vi "setEndTone.vi"(8 "error in (no error)":errorcluster, 10 "EndTone":refnum<class "ScriptEvent.lvclass">, 11 "SingleToneRamp.lvclass in":refnum<class "SingleToneRamp.lvclass">) -> (0 "error out":errorcluster, 3 "SingleToneRamp.lvclass out":refnum<class "SingleToneRamp.lvclass">)   [LabVIEW 2011, in "Tools.lvlib" / "Scripting.lvlib" / "SingleToneRamp.lvclass"]
uses:
  SingleToneRamp.lvclass
  ScriptEvent.lvclass
  SingleTone.lvclass
  SingleToneRamp.lvclass/SingleToneRamp.ctl
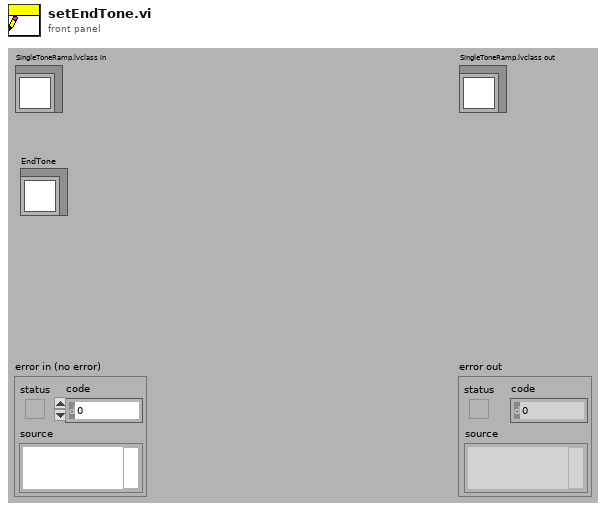
[diagram p1: front panel]
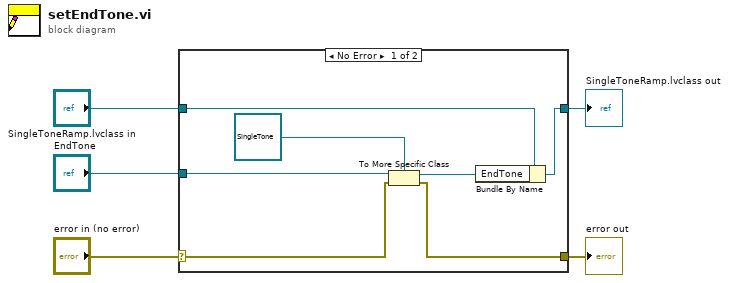
[diagram p0: block diagram]
diagram:
  n1 = case shown="No Error" "error in (no error)" {
    selector: "error in (no error)" -> [w7 w13]
    tunnel: [w6 w13] -> w4
    tunnel: [w12 w14] -> w2
    tunnel: "SingleToneRamp.lvclass in" -> [w11 w14]
    tunnel: "EndTone" -> [w10 _]
    frame No Error {
      n2 = To More Specific Class(target class=refnum<class "SingleTone.lvclass"> refnum ("Tools.lvlib:Scripting.lvlib:SingleTone.lvclass"), reference=w10, error in=w7) -> (specific class reference=w9:refnum<class "SingleTone.lvclass">, error out=w6:errorcluster)
      n3 = Bundle By Name(cluster=w11, "EndTone"=w9) -> (w12:refnum<class "SingleToneRamp.lvclass">)
    }
    frame Error {
    }
  }
  "error out" <- w4
  "SingleToneRamp.lvclass out" <- w2
